vi "Autonomous A2 left-deliverswitch-move out of way.vi"   [LabVIEW 2017]
uses:
  Framework/Robot Global Data.vi
types:
  T1 = typedef "Command Status Info.ctl" = cluster{"Name":string, "Status":T2, "notifier out":T3}
  T2 = typedef "Completion Status.ctl" = enum16{"Successful", "Aborted", "Incomplete"}
  T3 = typedef "Completion Notifier.ctl" = refnum<notifier>
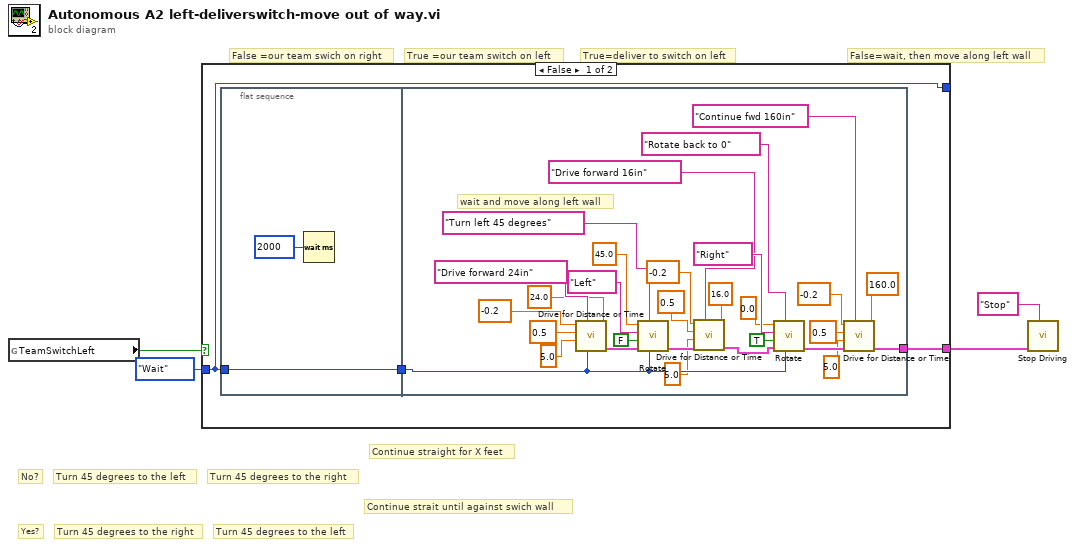
[diagram p0: block diagram]
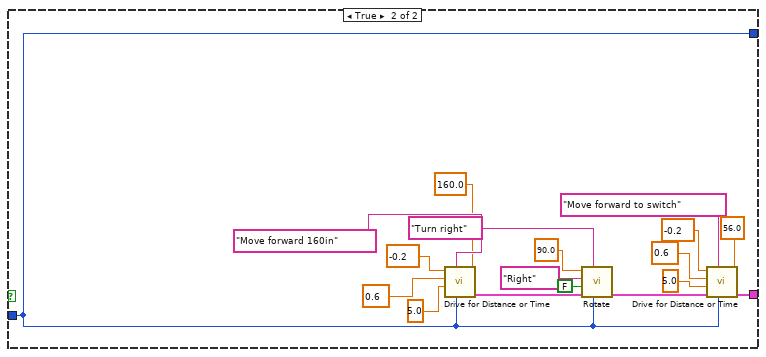
[diagram p2: hidden frame]
diagram:
  # "False=wait, then move along left wall"
  # "True=deliver to switch on left"
  # "False =our team swich on right"
  # "True =our team switch on left"
  # "Continue strait until against swich wall"
  # "Continue straight for X feet"
  # "Turn 45 degrees to the left"
  # "Turn 45 degrees to the right"
  # "Turn 45 degrees to the left"
  # "Turn 45 degrees to the right"
  # "No?"
  # "Yes?"
  n1 = global read "Robot Global Data.vi" "TeamSwitchLeft"() -> (w1:bool)
  n2 = case shown="False" w1 {
    tunnel: enum16{"Start", "Wait"}."Wait" ("Synchronication") -> [w7 w44]
    tunnel: [w5 w53] -> w2
    tunnel: [w7 w44] -> _
    frame False {
      n3 = flat-sequence {
        tunnel: w7 -> [w9]
        tunnel: [w9] -> w6
        tunnel: w6 -> [w29]
        tunnel: [w15] -> w5
        frame #0 {
          n4 = Wait (ms)(milliseconds to wait=u32 2000) -> ()  [unwired: 1 out]
        }
        frame #1 {
          # "wait and move along left wall"
          n5 = call "Drive for Distance or Time.vi"("Distance (inches)"=24.0, "Synchronication"=w29, "Description"="Drive forward 24in", "Seconds"=5.0, "Y-axis"=0.5 ("Right Speed"), "X-axis"=-0.2) -> ("Command Info Out"=w35:T1)  [unwired: 5 in]
          n6 = call "Rotate.vi"("Synchronication"=w29, "Description"="Turn left 45 degrees", "Command Info In"=w35, "Force Degrees"=FALSE, "Turn Direction"="Left" ("Direction"), "Degrees"=45.0) -> ("Command Info Out"=w24:T1)  [unwired: 5 in]
          n7 = call "Drive for Distance or Time.vi"("Distance (inches)"=16.0, "Description"="Drive forward 16in", "Command Info In"=w24, "Seconds"=5.0, "Y-axis"=0.5 ("Right Speed"), "X-axis"=-0.2) -> ("Command Info Out"=w23:T1)  [unwired: 5 in]
          n8 = call "Rotate.vi"("Synchronication"=w29, "Description"="Rotate back to 0", "Command Info In"=w23, "Force Degrees"=TRUE, "Turn Direction"="Right" ("Direction"), "Degrees"=0.0 ("Seconds")) -> ("Command Info Out"=w22:T1)  [unwired: 5 in]
          n9 = call "Drive for Distance or Time.vi"("Distance (inches)"=160.0, "Description"="Continue fwd 160in", "Command Info In"=w22, "Seconds"=5.0, "Y-axis"=0.5, "X-axis"=-0.2) -> ("Command Info Out"=w15:T1)  [unwired: 5 in]
        }
      }
    }
    frame True {
      n10 = call "Drive for Distance or Time.vi"("Distance (inches)"=160.0, "Synchronication"=w44, "Description"="Move forward 160in", "Seconds"=5.0, "Y-axis"=0.6 ("Right Speed"), "X-axis"=-0.2) -> ("Command Info Out"=w49:T1)  [unwired: 5 in]
      n11 = call "Rotate.vi"("Synchronication"=w44, "Description"="Turn right", "Command Info In"=w49, "Force Degrees"=FALSE, "Turn Direction"="Right" ("Direction"), "Degrees"=90.0 ("Seconds")) -> ("Command Info Out"=w48:T1)  [unwired: 5 in]
      n12 = call "Drive for Distance or Time.vi"("Distance (inches)"=56.0, "Synchronication"=w44, "Description"="Move forward to switch", "Command Info In"=w48, "Seconds"=5.0, "Y-axis"=0.6 ("Right Speed"), "X-axis"=-0.2) -> ("Command Info Out"=w53:T1)  [unwired: 4 in]
    }
  }
  n13 = call "Stop Driving.vi"("Description"="Stop", "Command Info In"=w2) -> ()  [unwired: 9 in, 1 out]
